vi "NI VeriStand - Save Macro.vi"(7 "error in (no error)":errorcluster, 9 "File path":path, 10 "MacroRecorder in":T1) -> (0 "error out":errorcluster, 3 "MacroRecorder out":T1)   [LabVIEW 2020, in "NI_VS MacroRecorderAPI.lvlib"]
doc: "Saves the current macro recording. You must use the Stop Macro Recording VI to stop recording before you call this VI. This VI creates a file of the type .nivsmacro. You can use the Macro Player VIs to load the file this VI creates and to play back the saved recording."
uses:
  <vilib>/NI VeriStand/Execution/MacroRecorder/NI_VS MacroRecorderAPI.lvlib
  <vilib>/NI VeriStand/Execution/MacroRecorder/MacroRecorderAPI.ctl
  NationalInstruments.VeriStand.ClientAPI
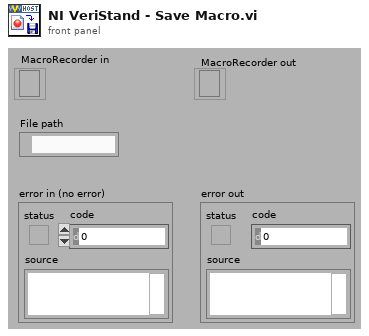
[diagram p1: front panel]
types:
  T1 = typedef "NI_VS MacroRecorderAPI.lvlib/MacroRecorderAPI.ctl" = refnum<k24>
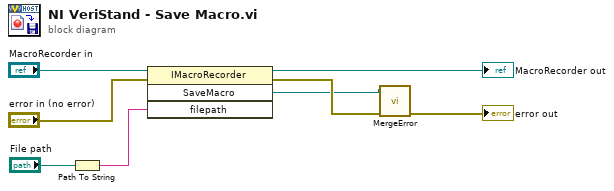
[diagram p0: block diagram]
diagram:
  n1 = Path To String(path="File path") -> (string=w2:string)
  n2 = invoke class="IMacroRecorder" method="SaveMacro"(reference="MacroRecorder in", error in="error in (no error)", "filepath"=w2) -> (reference out=→"MacroRecorder out":T1, error out=w6:errorcluster, "SaveMacro"=w1:refnum<k24>)  [unwired: 1 in, 1 out]
  n3 = call <vilib>:"MergeError.vi"("error in (no error)"=w6, "Error"=w1) -> ("error out"=→"error out":errorcluster)  [unwired: 9 out]
